vi "Set 135 LO via GPIB.vi"(3 "error in":T1, 4 "Hidden Controls (in)":T2 {"Prev Sampling Interval" format="%.1f"; "Prev Lo Setpoint" format="%.1f"; "Prev Hi Setpoint" format="%.1f"; "Prev Sensor Length" format="%.1f"; "Helium Level (cm)" format="%.1f"}, 5 "Configuration (in)":T3={"Sensor Length (cm)"=100.0, "Hi Setpoint (cm)"=80.0, "Lo Setpoint (cm)"=20.0, "Sampling Interval (min)"=1.0} {"Sampling Interval (min)" min=0 max=600 format="%.1f"; "Lo Setpoint (cm)" min=0 max=203.2 format="%.1f"; "Hi Setpoint (cm)" min=0 max=203.2 format="%.1f"; "Sensor Length (cm)" min=1 max=203.2 format="%.1f"}, 6 "GPIB Setup":cluster{"GPIB address":i16, "GPIB bus":i16}={"GPIB address"=1, "GPIB bus"=0}) -> (0 "error out":T1, 1 "Hidden Controls (out)":T2 {"Prev Sampling Interval" format="%.1f"; "Prev Lo Setpoint" format="%.1f"; "Prev Hi Setpoint" format="%.1f"; "Prev Sensor Length" format="%.1f"; "Helium Level (cm)" format="%.1f"}, 2 "Configuration (out)":T3={"Sensor Length (cm)"=100.0, "Hi Setpoint (cm)"=80.0, "Lo Setpoint (cm)"=20.0, "Sampling Interval (min)"=1.0} {"Sampling Interval (min)" min=0 max=600 format="%.1f"; "Lo Setpoint (cm)" min=0 max=203.2 format="%.1f"; "Hi Setpoint (cm)" min=0 max=203.2 format="%.1f"; "Sensor Length (cm)" min=1 max=203.2 format="%.1f"})   [LabVIEW 2019]
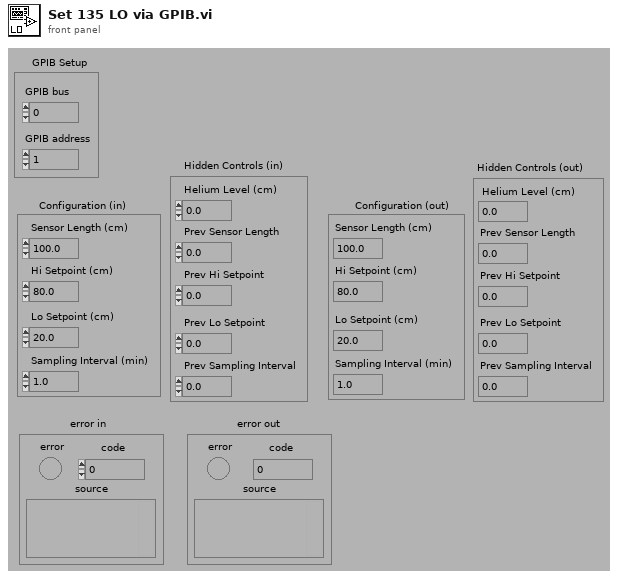
[diagram p1: front panel]
types:
  T1 = cluster{"error":bool, "code":i32, "source":string}
  T2 = cluster{"Helium Level (cm)":sgl, "Prev Sensor Length":sgl, "Prev Hi Setpoint":sgl, "Prev Lo Setpoint":sgl, "Prev Sampling Interval":sgl}
  T3 = cluster{"Sensor Length (cm)":sgl, "Hi Setpoint (cm)":sgl, "Lo Setpoint (cm)":sgl, "Sampling Interval (min)":sgl}
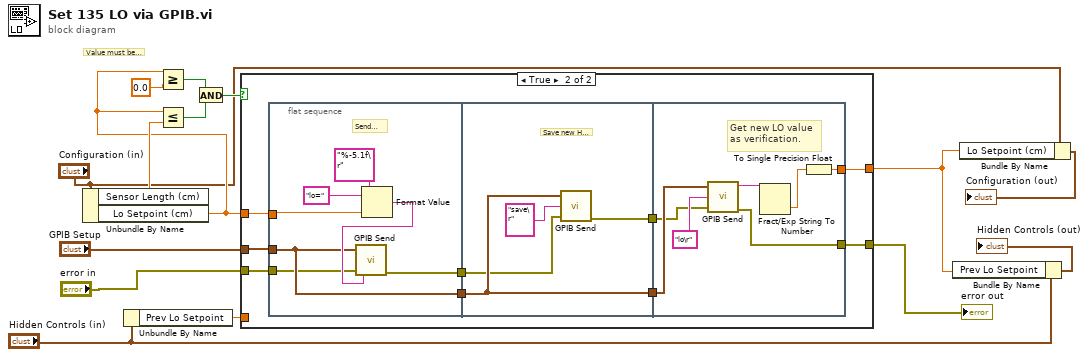
[diagram p0: block diagram]
diagram:
  # "Value must be >= 0 and <= length."
  n1 = Unbundle By Name("Configuration (in)") -> ("Sensor Length (cm)"=w14:sgl, "Lo Setpoint (cm)"=w13:sgl)
  n2 = Unbundle By Name("Hidden Controls (in)") -> ("Prev Lo Setpoint"=w8:sgl)
  n3 = Greater Or Equal?(x=w13, y=sgl 0.0) -> (x >= y?=w11:bool)
  n4 = Less Or Equal?(x=w13, y=w14) -> (x <= y?=w10:bool)
  n5 = And(x=w11, y=w10) -> (x .and. y?=w9:bool)
  n6 = case shown="True" w9 {
    tunnel: w13 -> [_ w26]
    tunnel: "GPIB Setup" -> [_ w25]
    tunnel: [w17 w24] -> w7
    tunnel: w8 -> [w17 _]
    tunnel: [w16 w19] -> w2
    tunnel: "error in" -> [w16 w18]
    frame False {
      # "New value out of range.\nNothing changed."
    }
    frame True {
      n7 = flat-sequence {
        tunnel: w25 -> [w29]
        tunnel: [w29] -> w23
        tunnel: w26 -> [w32]
        tunnel: [w28] -> w21
        tunnel: w18 -> [w27]
        tunnel: w23 -> [w36]
        tunnel: [w36] -> w22
        tunnel: w21 -> [w35]
        tunnel: [w34] -> w20
        tunnel: w22 -> [w41]
        tunnel: [w40] -> w24
        tunnel: w20 -> [w39]
        tunnel: [w38] -> w19
        frame #0 {
          # "Send new HI setting\nto instrument."
          n8 = Format Value(string ("")="lo=", format string="%-5.1f\r", value (0)=w32) -> (output string=w33:string)
          n9 = call "GPIB Send.vi"("GPIB Setup"=w29, "Input command"=w33, "error in"=w27) -> ("error out"=w28:T1)  [unwired: 3 out]
        }
        frame #1 {
          # "Save new HI setting."
          n10 = call "GPIB Send.vi"("GPIB Setup"=w36, "Input command"="save\r", "error in"=w35) -> ("error out"=w34:T1)  [unwired: 3 out]
        }
        frame #2 {
          # "Get new LO value\nas verification."
          n11 = call "GPIB Send.vi"("GPIB Setup"=w41, "Input command"="lo\r", "error in"=w39) -> ("Return string"=w43:string, "error out"=w38:T1)  [unwired: 2 out]
          n12 = Fract/Exp String To Number(string=w43) -> (number=w44:dbl)  [unwired: 3 in, 1 out]
          n13 = To Single Precision Float(number=w44) -> (single precision float=w40:sgl)
        }
      }
    }
  }
  "error out" <- w2
  n14 = Bundle By Name(cluster="Hidden Controls (in)", "Prev Lo Setpoint"=w7) -> (→"Hidden Controls (out)":T2)
  n15 = Bundle By Name(cluster="Configuration (in)", "Lo Setpoint (cm)"=w7) -> (→"Configuration (out)":T3)
